vi "Concatenador_tag_pdfSuper.vi"(0 "TAG_PDF_SPW":string, 5 "TAG_PDF_SPK":string, 7 "TAG_PDF_SKM":string, 9 "TAG_PDF_SKI":string, 11 "TAG_PDF_SKS":string) -> (8 "TAG_PDF_FINAL":string)   [LabVIEW 2019]
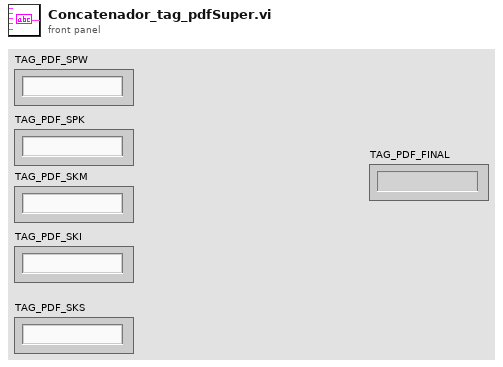
[diagram p1: front panel]
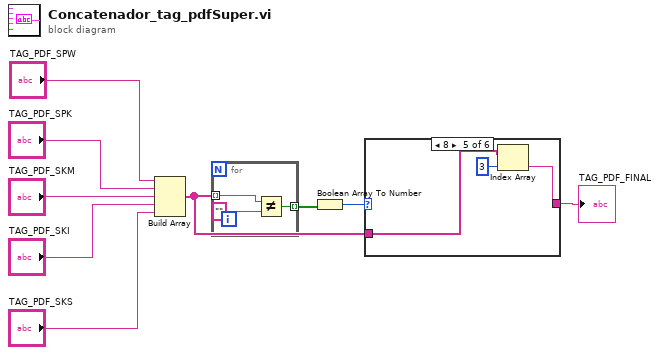
[diagram p0: block diagram]
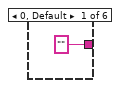
[diagram p2: hidden frame]
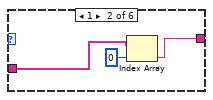
[diagram p3: hidden frame]
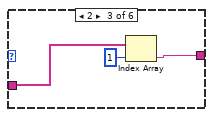
[diagram p4: hidden frame]
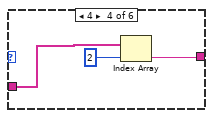
[diagram p5: hidden frame]
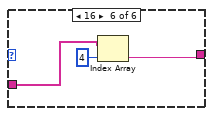
[diagram p6: hidden frame]
diagram:
  n1 = Build Array("TAG_PDF_SPW", "TAG_PDF_SPK", "TAG_PDF_SKM", "TAG_PDF_SKI", "TAG_PDF_SKS") -> (w1:string[])
  n2 = for {
    tunnel: w1 -> [w12] mode=indexing
    tunnel: [w10] -> w4 mode=indexing
    n3 = Not Equal?(x=w12, y="") -> (x != y?=w10:bool)
  }
  n4 = Boolean Array To Number(Boolean array=w4) -> (number=w3:u32)
  n5 = case shown="8" w3 {
    tunnel: ["" w14 w17 w20 w23 w26] -> w2
    tunnel: w1 -> [_ w16 w18 w21 w24 w27]
    frame 0, Default {
    }
    frame 1 {
      n6 = Index Array(array=w16, index=0) -> (element=w14:string)
    }
    frame 2 {
      n7 = Index Array(array=w18, index=1) -> (element=w17:string)
    }
    frame 4 {
      n8 = Index Array(array=w21, index=2) -> (element=w20:string)
    }
    frame 8 {
      n9 = Index Array(array=w24, index=3) -> (element=w23:string)
    }
    frame 16 {
      n10 = Index Array(array=w27, index=4) -> (element=w26:string)
    }
  }
  "TAG_PDF_FINAL" <- w2
